vi "Transcriptor LabVIEW to C code Engine 2.vi"(7 "vi path":path, 8 "Error In":errorcluster, 11 "Diagram in":refnum<vi>) -> (0 "Error Out":errorcluster, 1 "output cluster":T1, 2 "transcripted code":string, 3 "Diagram out":refnum<vi>)   [LabVIEW 2014]
uses:
  types/LabVIEW Universal Transcriptor Cluster.ctl
panel:
  out "FiringOrder":string[](array[string])
  # "0. create definitions (ClusterConstant)\n1. get all wires and create their declarations\n2. if wires are connected to control or constant assign value to them\n3. translate elements of diagram by firing order\n4. assign values to outputs"
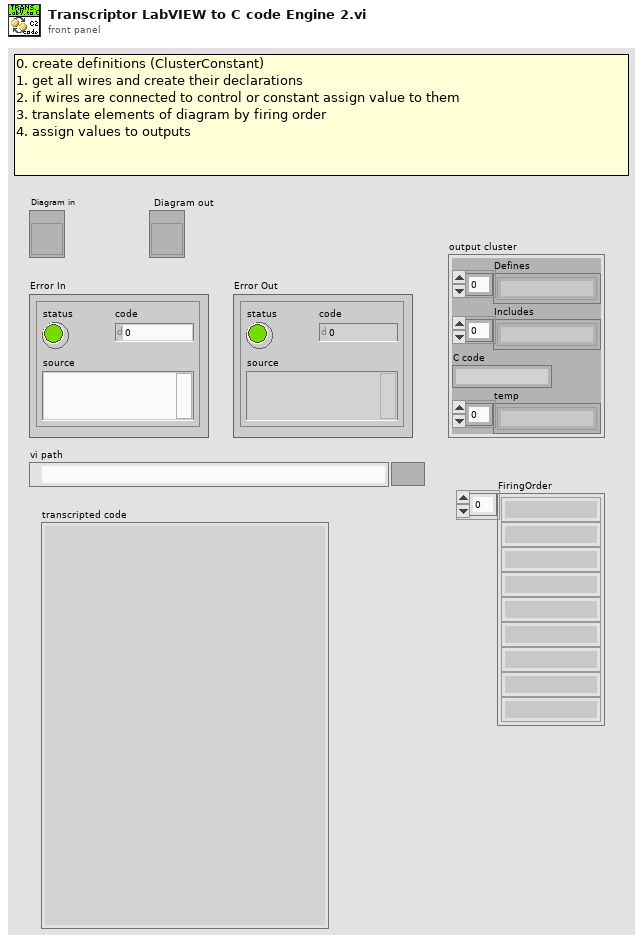
[diagram p1: front panel]
types:
  T1 = typedef "LabVIEW Universal Transcriptor Cluster.ctl" = cluster{"Defines":string[], "Includes":string[], "C code":string, "temp":string[]}
  T2 = cluster{"wire labels":string[], "wire terminals datatypes":string[][]}
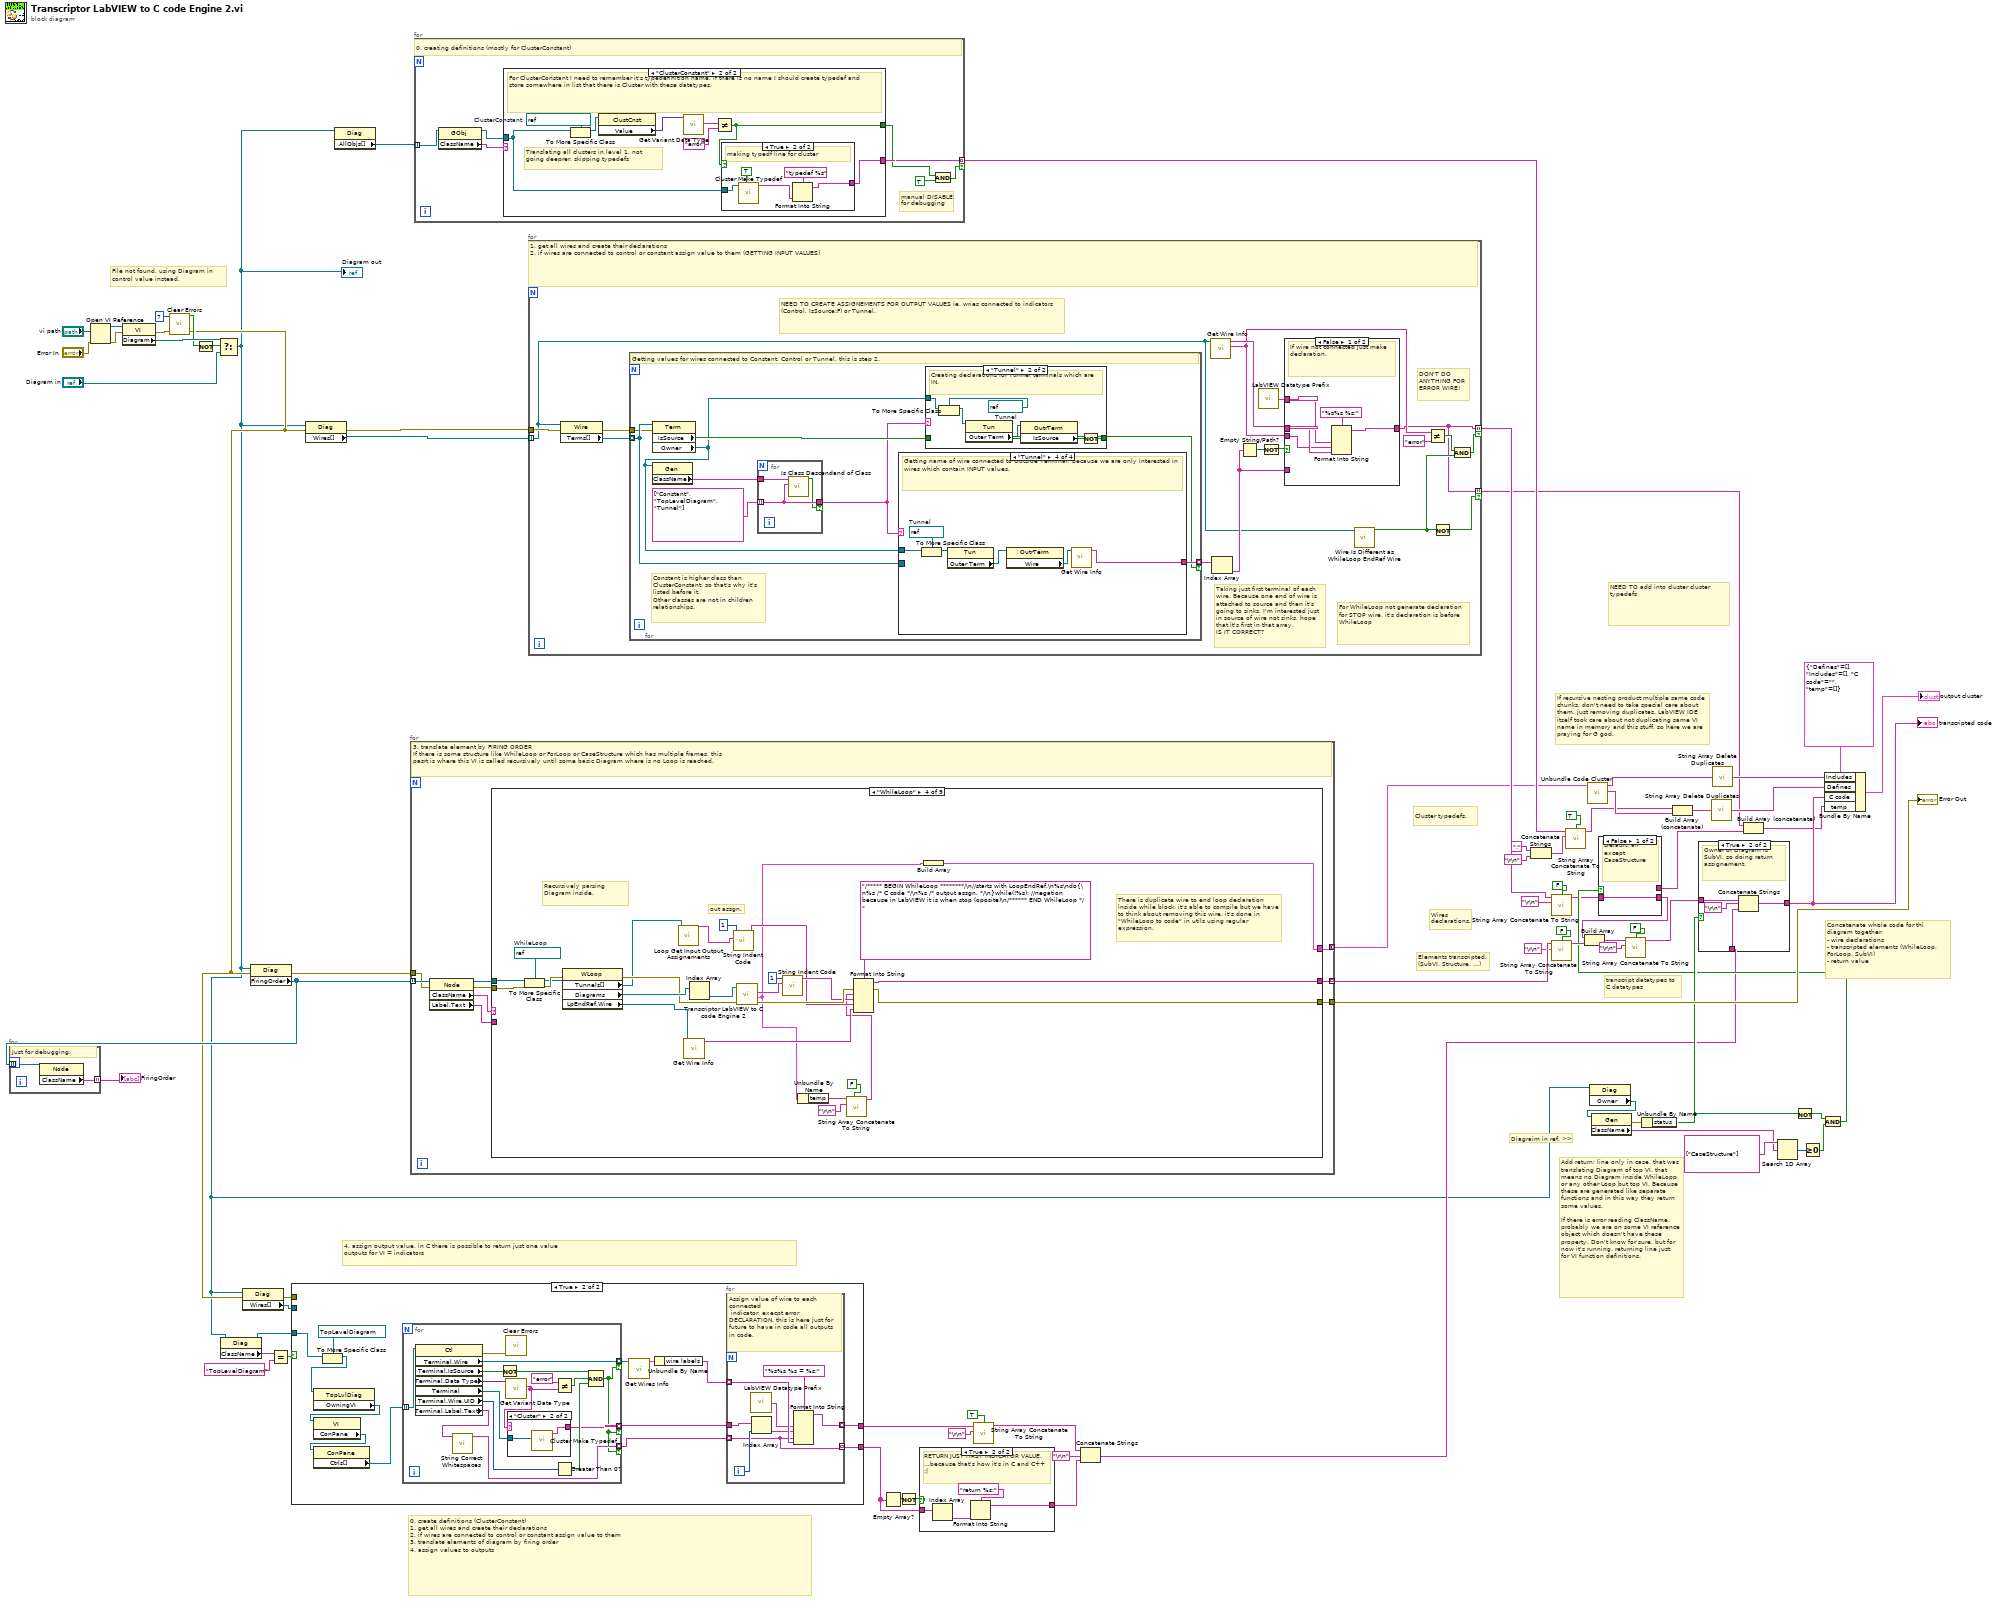
[diagram p0: block diagram]
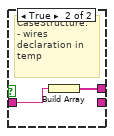
[diagram p7: hidden frame]
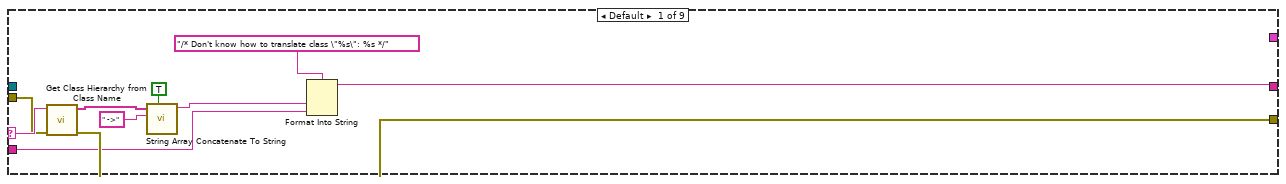
[diagram p9: hidden frame]
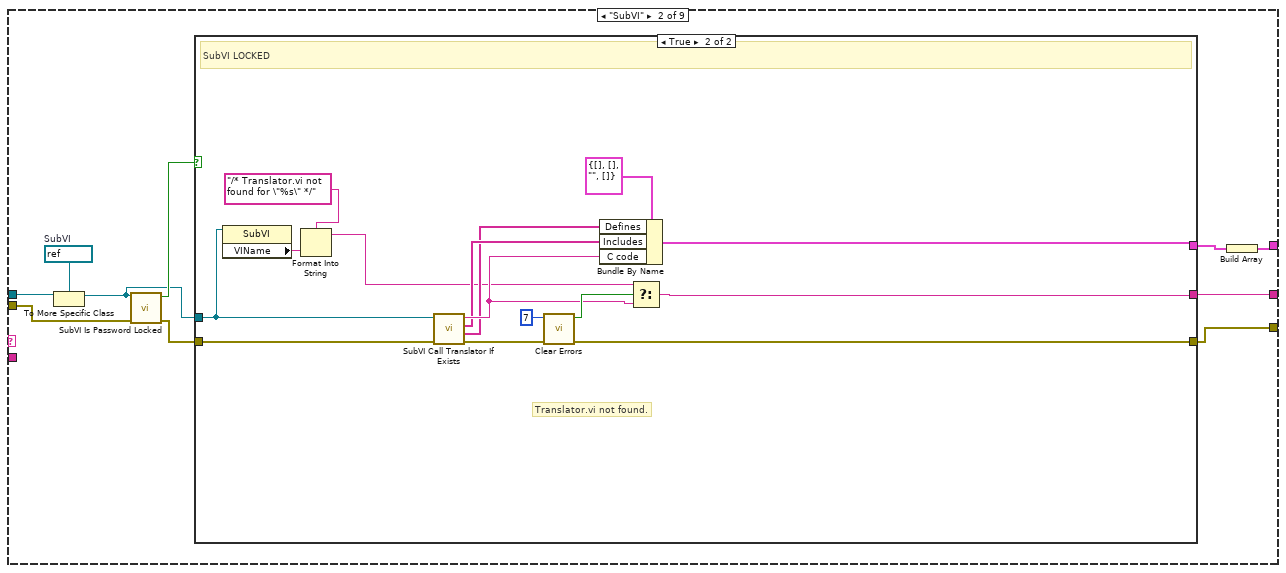
[diagram p10: hidden frame]
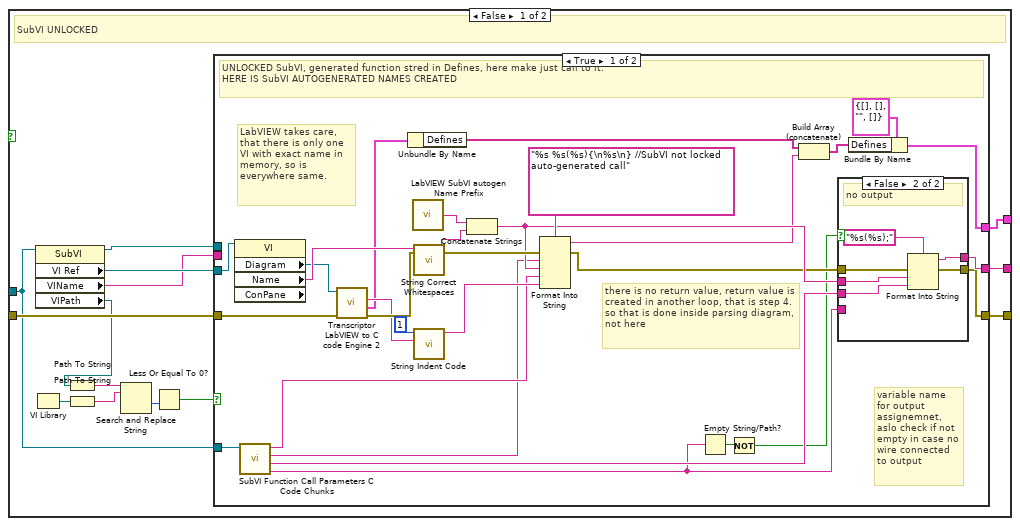
[diagram p11: hidden frame]
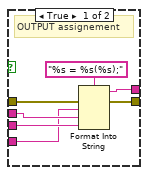
[diagram p12: hidden frame]
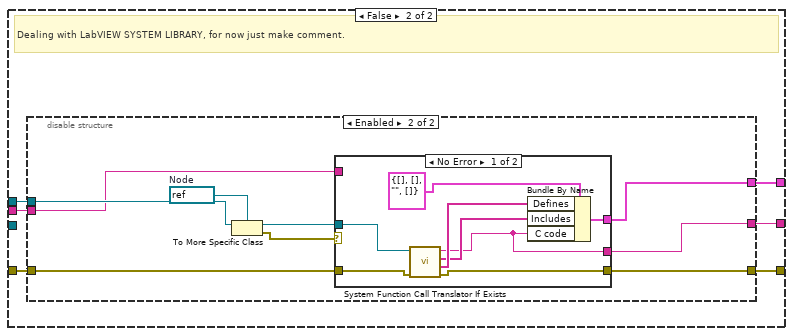
[diagram p13: hidden frame]
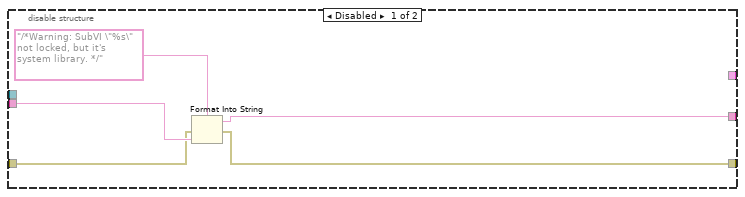
[diagram p14: hidden frame]
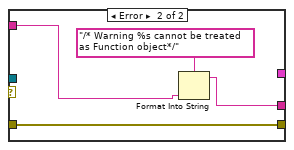
[diagram p15: hidden frame]
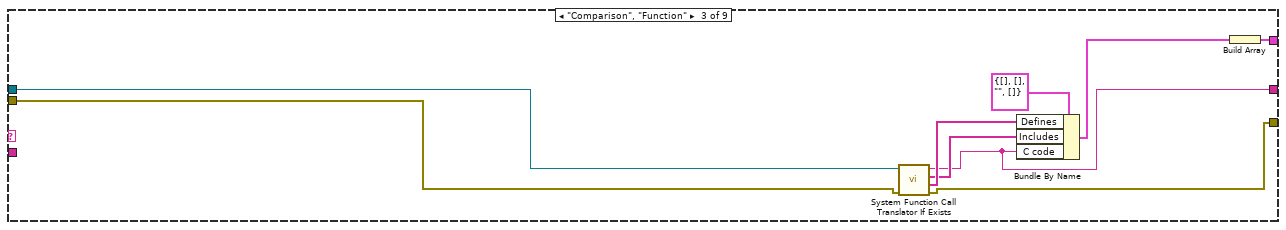
[diagram p16: hidden frame]
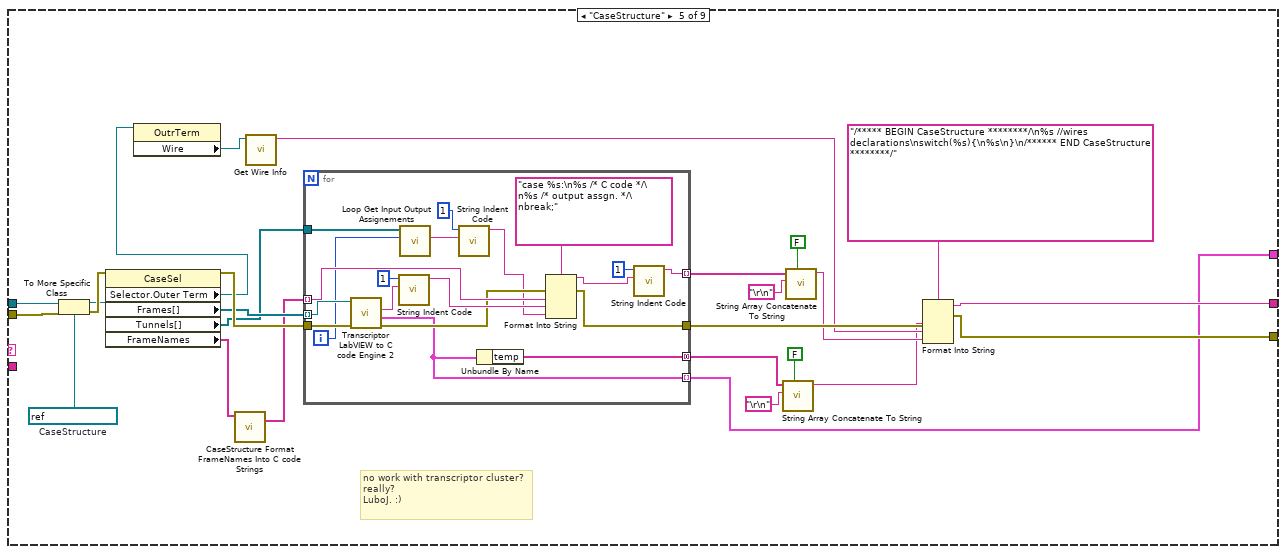
[diagram p17: hidden frame]
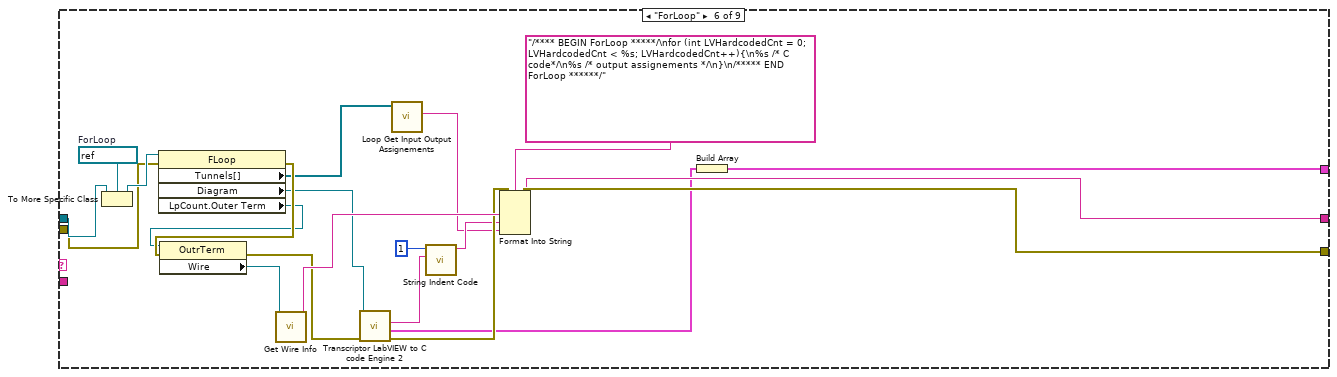
[diagram p18: hidden frame]
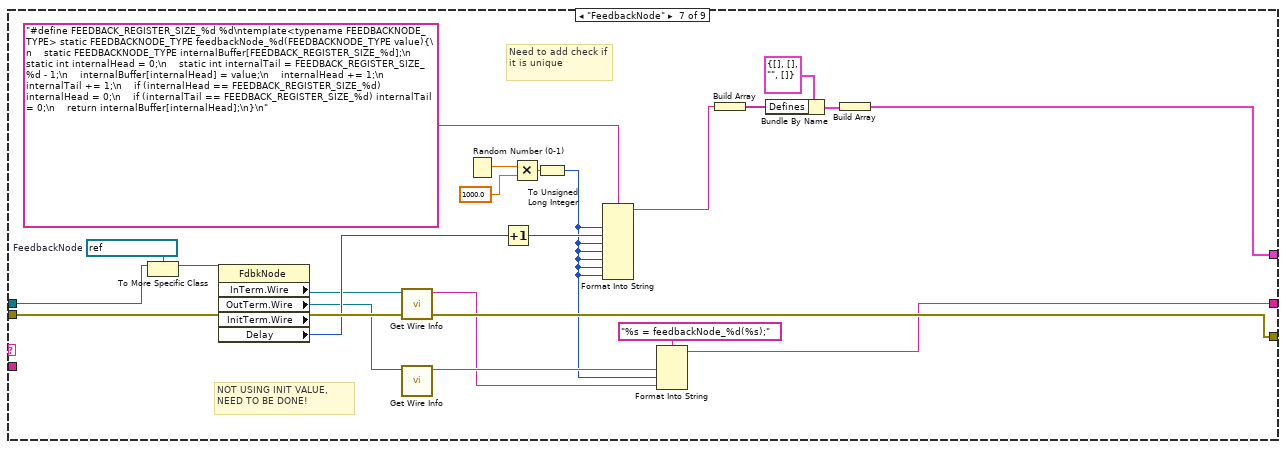
[diagram p19: hidden frame]
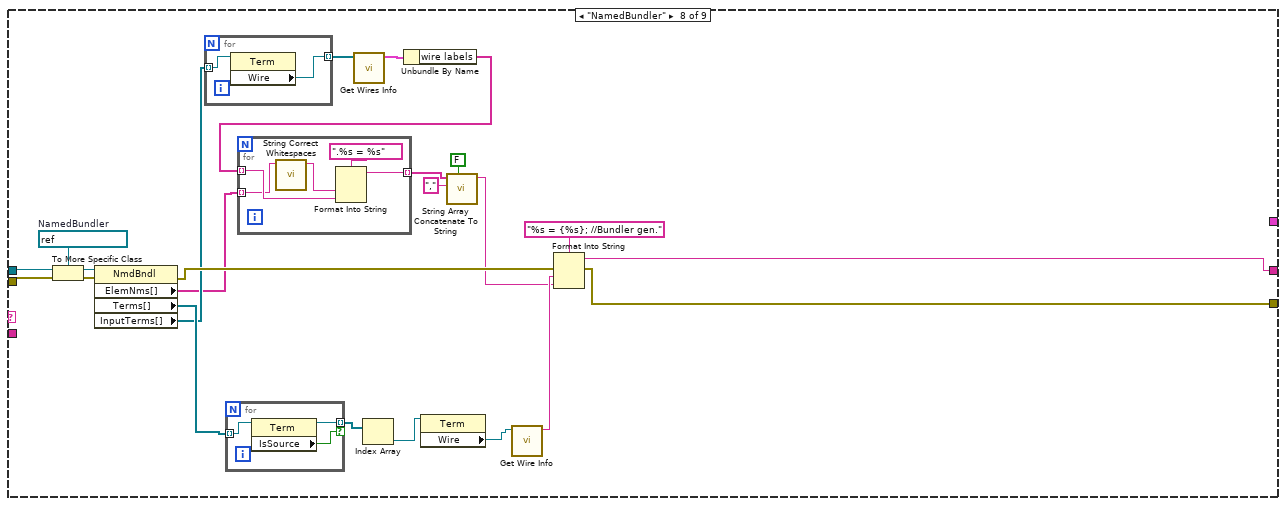
[diagram p20: hidden frame]
diagram:
  # "4. assign output value, in C there is possible to return just one value\noutputs for VI = indicators"
  # "Diagraim in ref. >>"
  # "Add return; line only in case, that was translating Diagram of top VI, that means no Diagram inside WhileLopp or any other Loop but top VI. Because these are generated like separate functions and in this way they return some values.\n\nIf there is error reading ClassName, probably we are on some VI reference object which doesn't have these property. Don't know for sure, but for now it's running, returning line just for VI function definitions."
  # "Concatenate whole code for thi diagram together:\n- wire declarations\n- transcripted elements (WhileLoop, ForLoop, SubVI)\n- return value"
  # "0. create definitions (ClusterConstant)\n1. get all wires and create their declarations\n2. if wires are connected to control or constant assign value to them\n3. translate elements of diagram by firing order\n4. assign values to outputs"
  # "If recursive nesting product multiple same code chunks, don't need to take special care about them, just removing duplicates, LabVIEW IDE itself took care about not duplicating same VI name in memory and this stuff, so here we are praying for G god."
  # "NEED TO add into cluster cluster typedefs"
  # "transcript datatypes to C datatypes"
  # "Elements transcripted.\n(SubVI, Structure, ...)"
  # "Wires declarations."
  # "Cluster typedefs."
  # "File not found, using Diagram in control value instead."
  n1 = Open VI Reference(vi path="vi path", error in (no error)="Error In") -> (vi reference=w20:refnum<vi>, error out=w74:errorcluster)  [unwired: 4 in]
  n2 = property class="VI"(reference=w20, error in=w74) -> (error out=w59:errorcluster, "Diagram"=w63:refnum<vi>)  [unwired: 1 out]
  n3 = call <vilib>:"Clear Errors.vi"("error in (no error)"=w59, "specific error code to clear (0: all)"=7) -> ("error out"=w42:errorcluster, "specific error cleared?"=w57:bool)  [unwired: 4 in]
  n4 = Not(x=w57) -> (.not. x?=w56:bool)
  n5 = Select(t=w63, s=w56, f="Diagram in") -> (s? t:f=w16:refnum<vi>)
  "Diagram out" <- w16
  n6 = property class="Diag"(reference=w16) -> (reference out=w15:refnum<vi>, "ClassName"=w18:string)  [unwired: 1 in, 1 out]
  n7 = property class="Diag"(reference=w16, error in=w42) -> (error out=w43:errorcluster, "Wires[]"=w44:refnum<vi>[])  [unwired: 1 out]
  n8 = property class="Diag"(reference=w16, error in=w42) -> (error out=w71:errorcluster, "FiringOrder"=w61:refnum<vi>[])  [unwired: 1 out]
  n9 = for {
    tunnel: w61 -> [w77] mode=indexing
    tunnel: [w76] -> w60 mode=indexing
    # "Just for debugging."
    n10 = property class="Node"(reference=w77) -> ("ClassName"=w76:string)  [unwired: 1 in, 2 out]
  }
  "FiringOrder" <- w60
  n11 = Equal?(x=w18, y="TopLevelDiagram" ("Parent ClassName")) -> (x = y?=w17:bool)
  n12 = case shown="True" w17 {
    tunnel: w44 -> [_ _]
    tunnel: w43 -> [_ _]
    tunnel: [_ w90] -> w39
    tunnel: [_ w89] -> w23
    tunnel: w15 -> [_ w87]
    frame False {
    }
    frame True {
      n13 = To More Specific Class(target class=refnum<vi> refnum, reference=w87) -> (specific class reference=w86:refnum<vi>)  [unwired: 1 in, 1 out]
      n14 = property class="TopLvlDiag"(reference=w86) -> ("OwningVI"=w85:refnum<vi>)  [unwired: 1 in, 2 out]
      n15 = property class="VI"(reference=w85) -> ("ConPane"=w84:refnum<vi>)  [unwired: 1 in, 2 out]
      n16 = property class="ConPane"(reference=w84) -> ("Ctrls[]"=w83:refnum<vi>[])  [unwired: 1 in, 2 out]
      n17 = for {
        tunnel: w83 -> [w106] mode=indexing
        tunnel: [w93] -> w82 mode=indexing if=w91
        tunnel: [w95] -> w81 mode=indexing if=w91
        tunnel: [w92] -> w80 mode=indexing if=w91
        n18 = property class="Ctl"(reference=w106) -> (error out=w105:errorcluster, "Terminal.Wire"=w92:refnum<vi>, "Terminal.IsSource"=w104:bool, "Terminal.Data Type"=w103:variant, "Terminal"=w100:refnum<vi>, "Terminal.Wire.UID"=w99:i32, "Terminal.Label.Text"=w94:string)  [unwired: 1 in, 1 out]
        n19 = call "String Correct Whitespaces.vi"("String in"=w94) -> ("String out"=w93:string)  [unwired: 10 in]
        n20 = Not(x=w104) -> (.not. x?=w98:bool)
        n21 = call <vilib>:"Clear Errors.vi"("error in (no error)"=w105) -> ()  [unwired: 5 in, 2 out]
        n22 = call "Get Variant Data Type.vi"("Variant in"=w103) -> ("first data type"=w101:string)  [unwired: 9 in, 1 out]
        n23 = case shown="\"Cluster\"" w101 {
          selector: w101 -> [w107 _]
          tunnel: [w107 w109] -> w95
          tunnel: w100 -> [_ w108]
          frame Default {
          }
          frame "Cluster" {
            n24 = call "Cluster Make Typedef.vi"("Terminal in"=w108) -> ("String"=w109:string)  [unwired: 10 in]
          }
        }
        n25 = Not Equal?(x="error", y=w101) -> (x != y?=w97:bool)
        n26 = Greater Than 0?(x=w99) -> (x > 0?=w96:bool)
        n27 = Compound Arithmetic op=AND(w98, w97, w96) -> (w91:bool)
      }
      n28 = call "Get Wires Info.vi"("connected\nwires refs."=w80) -> ("output cluster 2"=w79:T2)  [unwired: 10 in]
      n29 = Unbundle By Name(w79) -> ("wire labels"=w78:string[])
      n30 = for {
        tunnel: w82 -> [w110] mode=indexing
        tunnel: w78 -> [w115] mode=indexing
        tunnel: [w116] -> w90 mode=indexing
        tunnel: w81 -> [w113]
        tunnel: [w110] -> w89 mode=indexing
        i -> [w114]
        # "Assign value of wire to each connected\n indicator, execpt error\nDECLARATION, this is here just for future to have in code all outputs in code."
        n31 = call "LabVIEW Datatype Prefix.vi"() -> ("datatype prefix"=w111:string)
        n32 = Index Array(array=w113, index=w114) -> (element=w112:string)
        n33 = Format Into String(format string="%s%s %s = %s;", w111, w112, w110, w115) -> (resulting string=w116:string)  [unwired: 2 in, 1 out]
      }
    }
  }
  n34 = property class="Diag"(reference=w16, error in=w42) -> (error out=w72:errorcluster, "Wires[]"=w73:refnum<vi>[])  [unwired: 1 out]
  n35 = property class="Diag"(reference=w16) -> ("AllObjs[]"=w11:refnum<vi>[])  [unwired: 1 in, 2 out]
  n36 = for {
    tunnel: w61 -> [w126] mode=indexing
    tunnel: w71 -> [w124]
    tunnel: [w122] -> w70 mode=indexing
    tunnel: [w120] -> w32
    tunnel: [w119] -> w33 mode=concatenating
    # "3. translate element by FIRING ORDER\nIf there is some structure like WhileLoop or ForLoop or CaseStructure which has multiple frames, this\npasrt is where this VI is called recursively until some basic Diagram where is no Loop is reached."
    n37 = property class="Node"(reference=w126, error in=w124) -> (reference out=w123:refnum<vi>, error out=w121:errorcluster, "ClassName"=w125:string, "Label.Text"=w118:string)
    n38 = case shown="\"WhileLoop\"" w125 {
      selector: w125 -> [w134 _ _ _ _ _ _ _ _]
      tunnel: w123 -> [_ w146 w256 w284 w292 w350 w371 w395 w425]
      tunnel: [w135 w142 w253 w276 w305 w340 w359 w382 w406] -> w122
      tunnel: w121 -> [w129 w141 w257 w280 w308 w347 w372 w394 w424]
      tunnel: [w128 w139 w250 w274 w303 w341 w372 w380 w418] -> w120
      tunnel: [_ w137 w252 w263 w285 w330 w366 _ _] -> w119
      tunnel: w118 -> [w127 _ _ _ _ _ _ _ _]
      frame Default {
        n39 = call <vilib>:"Get Class Hierarchy from Class Name.vi"("error in (no error)"=w129, "Class Name"=w134) -> ("error out"=w128:errorcluster, "Class Hierarchy"=w132:string[])  [unwired: 8 in]
        n40 = call "String Array Concatenate To String.vi"("insert last delimiter?"=TRUE, "Delimiter char"=" ->", "Array String In"=w132) -> ("String"=w130:string)  [unwired: 8 in]
        n41 = Format Into String(format string="/* Don't know how to translate class \"%s\": %s */", w130, w127) -> (resulting string=w135:string)  [unwired: 2 in, 1 out]
      }
      frame "SubVI" {
        w145 = refnum<vi> refnum  # SubVI
        n42 = To More Specific Class(target class=w145, reference=w146) -> (specific class reference=w143:refnum<vi>)  [unwired: 1 in, 1 out]
        n43 = call "SubVI Is Password Locked.vi"("Error In"=w141, "SubVI ref"=w143) -> ("Error Out"=w140:errorcluster, "isPasswordLocked?"=w144:bool)  [unwired: 8 in]
        n44 = case shown="True" w144 {
          tunnel: w143 -> [w148 w239]
          tunnel: [w158 w245] -> w142
          tunnel: w140 -> [w160 w244]
          tunnel: [w157 w243] -> w139
          tunnel: [w149 w235] -> w138
          frame False {
            # "SubVI UNLOCKED"
            n45 = VI Library() -> (path=w154:path)
            n46 = property class="SubVI"(reference=w148) -> (reference out=w147:refnum<vi>, "VI Ref"=w159:refnum<vi>, "VIName"=w156:string, "VIPath"=w155:path)  [unwired: 1 in, 1 out]
            n47 = Path To String(path=w155) -> (string=w153:string)
            n48 = Path To String(path=w154) -> (string=w152:string)
            n49 = Search and Replace String(input string=w153, search string=w152) -> (number of replacements=w151:i32)  [unwired: 6 in, 3 out]
            n50 = Less Or Equal To 0?(x=w151) -> (x <= 0?=w150:bool)
            n51 = case shown="True" w150 {
              tunnel: w160 -> [w188 w205]
              tunnel: w159 -> [w172 _]
              tunnel: [w186 w207] -> w158
              tunnel: [w174 w204] -> w157
              tunnel: w156 -> [_ w206]
              tunnel: [w187 w202] -> w149
              tunnel: w148 -> [w170 _]
              tunnel: w147 -> [_ w203]
              frame True {
                # "variable name for output assignemnet, aslo check if not empty in case no wire connected to output"
                # "there is no return value, return value is created in another loop, that is step 4.\nso that is done inside parsing diagram, not here"
                # "LabVIEW takes care, that there is only one VI with exact name in memory, so is everywhere same."
                # "UNLOCKED SubVI, generated function stred in Defines, here make just call to it.\nHERE IS SubVI AUTOGENERATED NAMES CREATED"
                n52 = property class="VI" props=["Diagram", "Name", "ConPane"](reference=w172) -> ("Diagram"=w173:refnum<vi>, "Name"=w183:string)  [unwired: 1 in, 3 out]
                n53 = call "SubVI Function Call Parameters C Code Chunks.vi"("SubVI Refnum"=w170) -> ("SubVI output variable name"=w166:string, "SubVI func. params  declaration"=w168:string, "return datatype"=w164:string, "SubVI func. call params"=w169:string)  [unwired: 6 in, 1 out]
                n54 = call "Transcriptor LabVIEW to C code Engine 2.vi"("Error In"=w188, "Diagram in"=w173) -> ("Error Out"=w184:errorcluster, "output cluster"=w163:T1, "transcripted code"=w182:string)  [unwired: 6 in, 1 out]
                n55 = Unbundle By Name(w163) -> ("Defines"=w162:string[])
                n56 = call "LabVIEW SubVI autogen Name Prefix.vi"() -> ("datatype prefix"=w180:string)
                n57 = call "String Correct Whitespaces.vi"("String in"=w183) -> ("String out"=w179:string)  [unwired: 10 in]
                n58 = call "String Indent Code.vi"("complete code"=w182, "actual nested level"=1) -> ("indented code"=w171:string)  [unwired: 9 in]
                n59 = Concatenate Strings(w180, w179) -> (w178:string)
                n60 = Format Into String(format string="%s %s(%s){\n%s\n} //SubVI not locked auto-generated call", error in=w184, w164, w178, w169, w171) -> (resulting string=w176:string, error out=w175:errorcluster)  [unwired: 1 in]
                n61 = Empty String/Path?(string/path=w166) -> (empty?=w167:bool)
                n62 = Not(x=w167) -> (.not. x?=w165:bool)
                n63 = Build Array (concatenate)(w162, w176) -> (w177:string[])
                n64 = case shown="False" w165 {
                  tunnel: [w195 w201] -> w186
                  tunnel: w178 -> [w193 w199]
                  tunnel: w175 -> [w192 w198]
                  tunnel: [w191 w197] -> w174
                  tunnel: w168 -> [w190 w196]
                  tunnel: w166 -> [w189 _]
                  frame True {
                    # "OUTPUT assignement"
                    n65 = Format Into String(format string="%s = %s(%s);", error in=w192, w189, w193, w190) -> (resulting string=w195:string, error out=w191:errorcluster)  [unwired: 1 in]
                  }
                  frame False {
                    # "no output"
                    n66 = Format Into String(format string="%s(%s);", error in=w198, w199, w196) -> (resulting string=w201:string, error out=w197:errorcluster)  [unwired: 1 in]
                  }
                }
                n67 = Bundle By Name(cluster=T1 {"Defines"=[], "Includes"=[], "C code"="", "temp"=[]} ("input cluster"), "Defines"=w177) -> (w187:T1)
              }
              frame False {
                # "Dealing with LabVIEW SYSTEM LIBRARY, for now just make comment."
                n68 = disable-structure shown="Enabled" {
                  disable-tunnel: [w211 w216] -> w207
                  disable-tunnel: w206 -> [w210 w213]
                  disable-tunnel: w205 -> [w209 w215]
                  disable-tunnel: [w208 w221] -> w204
                  disable-tunnel: w203 -> [_ w220]
                  disable-tunnel: [_ w217] -> w202
                  frame Disabled {
                    n69 = Format Into String(format string="/*Warning: SubVI \"%s\" not locked, but it's system library. */", error in=w209, w210) -> (resulting string=w211:string, error out=w208:errorcluster)  [unwired: 1 in]
                  }
                  frame Enabled {
                    w219 = refnum<vi> refnum  # Node
                    n70 = To More Specific Class(target class=w219, reference=w220) -> (specific class reference=w218:refnum<vi>, error out=w214:errorcluster)  [unwired: 1 in]
                    n71 = case shown="No Error" w214 {
                      tunnel: [w229 w233] -> w221
                      tunnel: w218 -> [w228 _]
                      tunnel: [w225 _] -> w217
                      tunnel: [w224 w230] -> w216
                      tunnel: w215 -> [w223 w233]
                      tunnel: w213 -> [_ w231]
                      frame No Error {
                        n72 = call "System Function Call Translator If Exists.vi"("Error In"=w223, "Node Refnum"=w228) -> ("Error Out"=w229:errorcluster, "Defines"=w227:string[], "Includes"=w226:string[], "Replaced Code"=w224:string)  [unwired: 6 in]
                        n73 = Bundle By Name(cluster=T1 {"Defines"=[], "Includes"=[], "C code"="", "temp"=[]} ("input cluster"), "Defines"=w227, "Includes"=w226, "C code"=w224) -> (w225:T1)
                      }
                      frame Error {
                        n74 = Format Into String(format string="/* Warning %s cannot be treated as Function object*/" ("Replaced Code"), w231) -> (resulting string=w230:string)  [unwired: 2 in, 1 out]
                      }
                    }
                  }
                }
              }
            }
          }
          frame True {
            # "Translator.vi not found."
            # "SubVI LOCKED"
            n75 = property class="SubVI"(reference=w239) -> ("VIName"=w238:string)  [unwired: 1 in, 2 out]
            n76 = Format Into String(format string="/* Translator.vi not found for \"%s\" */" ("t"), w238) -> (resulting string=w236:string)  [unwired: 2 in, 1 out]
            n77 = call "SubVI Call Translator If Exists.vi"("Error In"=w244, "SubVI Refnum"=w239) -> ("Error Out"=w248:errorcluster, "Defines"=w240:string[], "Includes"=w241:string[], "Replaced Code"=w242:string)  [unwired: 6 in]
            n78 = call <vilib>:"Clear Errors.vi"("error in (no error)"=w248, "specific error code to clear (0: all)"=7) -> ("error out"=w243:errorcluster, "specific error cleared?"=w246:bool)  [unwired: 4 in]
            n79 = Bundle By Name(cluster=T1 {"Defines"=[], "Includes"=[], "C code"="", "temp"=[]} ("input cluster"), "Defines"=w240, "Includes"=w241, "C code"=w242) -> (w235:T1)
            n80 = Select(t=w236, s=w246, f=w242) -> (s? t:f=w245:string)
          }
        }
        n81 = Build Array(w138) -> (w137:T1[])
      }
      frame "Comparison", "Function" {
        n82 = call "System Function Call Translator If Exists.vi"("Error In"=w257, "Node Refnum"=w256) -> ("Error Out"=w250:errorcluster, "Defines"=w255:string[], "Includes"=w254:string[], "Replaced Code"=w253:string)  [unwired: 6 in]
        n83 = Bundle By Name(cluster=T1 {"Defines"=[], "Includes"=[], "C code"="", "temp"=[]} ("input cluster"), "Defines"=w255, "Includes"=w254, "C code"=w253) -> (w251:T1)
        n84 = Build Array(w251) -> (w252:T1[])
      }
      frame "WhileLoop" {
        w283 = refnum<vi> refnum  # WhileLoop
        # "out assgn."
        # "There is duplicate wire to end loop declaration inside while block, it's able to compile but we have to think about removing this wire, it's done in \"WhileLoop to code\" in utils using regular expression."
        # "Recursively parsing Diagram inside."
        n85 = To More Specific Class(target class=w283, reference=w284, error in=w280) -> (specific class reference=w273:refnum<vi>, error out=w282:errorcluster)
        n86 = property class="WLoop"(reference=w273, error in=w282) -> (error out=w279:errorcluster, "Tunnels[]"=w268:refnum<vi>[], "Diagrams"=w281:refnum<vi>[], "LpEndRef.Wire"=w272:refnum<vi>)  [unwired: 1 out]
        n87 = call "Loop Get Input Output Assignements.vi"("Loop Tunnels[]"=w268) -> ("Output assignements"=w265:string)  [unwired: 9 in, 1 out]
        n88 = call "Get Wire Info.vi"("Wire"=w272) -> ("wire label"=w267:string)  [unwired: 9 in, 1 out]
        n89 = Index Array(array=w281) -> (element=w278:refnum<vi>)  [unwired: 1 in]
        n90 = call "String Indent Code.vi"("complete code"=w265, "actual nested level"=1) -> ("indented code"=w264:string)  [unwired: 9 in]
        n91 = call "Transcriptor LabVIEW to C code Engine 2.vi"("Error In"=w279, "Diagram in"=w278) -> ("Error Out"=w275:errorcluster, "output cluster"=w262:T1, "transcripted code"=w271:string)  [unwired: 6 in, 1 out]
        n92 = call "String Indent Code.vi"("complete code"=w271, "actual nested level"=1) -> ("indented code"=w269:string)  [unwired: 9 in]
        n93 = Unbundle By Name(w262) -> ("temp"=w261:string[])
        n94 = call "String Array Concatenate To String.vi"("insert last delimiter?"=FALSE, "Delimiter char"="\r\n", "Array String In"=w261) -> ("String"=w258:string)  [unwired: 8 in]
        n95 = Format Into String(format string="/***** BEGIN WhileLoop ********/\n//starts with LoopEndRef.\n%s\ndo{\n%s /* C code */\n%s /* output assgn. */\n}while(!%s); //negation because in LabVIEW it is when stop (oposite)\n/****** END WhileLoop */", error in=w275, w258, w269, w264, w267) -> (resulting string=w276:string, error out=w274:errorcluster)  [unwired: 1 in]
        n96 = Build Array(w262) -> (w263:T1[])
      }
      frame "CaseStructure" {
        w310 = refnum<vi> refnum  # CaseStructure
        # "no work with transcriptor cluster? really?\nLuboJ. :)"
        n97 = To More Specific Class(target class=w310, reference=w292, error in=w308) -> (specific class reference=w302:refnum<vi>, error out=w309:errorcluster)
        n98 = property class="CaseSel"(reference=w302, error in=w309) -> (error out=w307:errorcluster, "Selector.Outer Term"=w300:refnum<vi>, "Frames[]"=w301:refnum<vi>[], "Tunnels[]"=w293:refnum<vi>[], "FrameNames"=w290:string[])  [unwired: 1 out]
        n99 = property class="OutrTerm"(reference=w300) -> ("Wire"=w299:refnum<vi>)  [unwired: 1 in, 2 out]
        n100 = call "CaseStructure Format FrameNames Into C code Strings.vi"("FrameNames in"=w290) -> ("c code cases names"=w291:string[])  [unwired: 10 in]
        n101 = call "Get Wire Info.vi"("Wire"=w299) -> ("wire label"=w298:string)  [unwired: 9 in, 1 out]
        n102 = for {
          tunnel: w307 -> [w329]
          tunnel: [w321] -> w304
          tunnel: w301 -> [w328] mode=indexing
          tunnel: w291 -> [w324] mode=indexing
          tunnel: [w319] -> w295 mode=indexing
          tunnel: w293 -> [w316]
          tunnel: [w312] -> w286 mode=concatenating
          tunnel: [w311] -> w285 mode=indexing
          i -> [w317]
          n103 = call "Transcriptor LabVIEW to C code Engine 2.vi"("Error In"=w329, "Diagram in"=w328) -> ("Error Out"=w322:errorcluster, "output cluster"=w311:T1, "transcripted code"=w326:string)  [unwired: 6 in, 1 out]
          n104 = call "String Indent Code.vi"("complete code"=w326, "actual nested level"=1) -> ("indented code"=w325:string)  [unwired: 9 in]
          n105 = call "Loop Get Input Output Assignements.vi"("Inside Terms[] offset"=w317, "Loop Tunnels[]"=w316) -> ("Output assignements"=w314:string)  [unwired: 8 in, 1 out]
          n106 = call "String Indent Code.vi"("complete code"=w314, "actual nested level"=1) -> ("indented code"=w313:string)  [unwired: 9 in]
          n107 = Unbundle By Name(w311) -> ("temp"=w312:string[])
          n108 = Format Into String(format string="case %s:\n%s /* C code */\n%s /* output assgn. */\nbreak;", error in=w322, w324, w325, w313) -> (resulting string=w318:string, error out=w321:errorcluster)  [unwired: 1 in]
          n109 = call "String Indent Code.vi"("complete code"=w318, "actual nested level"=1) -> ("indented code"=w319:string)  [unwired: 9 in]
        }
        n110 = call "String Array Concatenate To String.vi"("insert last delimiter?"=FALSE, "Delimiter char"="\r\n", "Array String In"=w286) -> ("String"=w287:string)  [unwired: 8 in]
        n111 = call "String Array Concatenate To String.vi"("insert last delimiter?"=FALSE, "Delimiter char"="\r\n", "Array String In"=w295) -> ("String"=w294:string)  [unwired: 8 in]
        n112 = Format Into String(format string="/***** BEGIN CaseStructure ********/\n%s //wires declarations\nswitch(%s){\n%s\n}\n/****** END CaseStructure ********/", error in=w304, w287, w298, w294) -> (resulting string=w305:string, error out=w303:errorcluster)  [unwired: 1 in]
      }
      frame "ForLoop" {
        w349 = refnum<vi> refnum  # ForLoop
        n113 = To More Specific Class(target class=w349, reference=w350) -> (specific class reference=w348:refnum<vi>)  [unwired: 1 in, 1 out]
        n114 = property class="FLoop"(reference=w348, error in=w347) -> (error out=w346:errorcluster, "Tunnels[]"=w333:refnum<vi>[], "Diagram"=w339:refnum<vi>, "LpCount.Outer Term"=w345:refnum<vi>)  [unwired: 1 out]
        n115 = property class="OutrTerm"(reference=w345, error in=w346) -> (error out=w338:errorcluster, "Wire"=w344:refnum<vi>)  [unwired: 1 out]
        n116 = call "Get Wire Info.vi"("Wire"=w344) -> ("wire label"=w342:string)  [unwired: 9 in, 1 out]
        n117 = call "Transcriptor LabVIEW to C code Engine 2.vi"("Error In"=w338, "Diagram in"=w339) -> ("Error Out"=w337:errorcluster, "output cluster"=w331:T1, "transcripted code"=w336:string)  [unwired: 6 in, 1 out]
        n118 = call "Loop Get Input Output Assignements.vi"("Loop Tunnels[]"=w333) -> ("Output assignements"=w332:string)  [unwired: 9 in, 1 out]
        n119 = call "String Indent Code.vi"("complete code"=w336, "actual nested level"=1) -> ("indented code"=w334:string)  [unwired: 9 in]
        n120 = Format Into String(format string="/**** BEGIN ForLoop *****/\nfor (int LVHardcodedCnt = 0;  LVHardcodedCnt < %s; LVHardcodedCnt++){\n%s /* C code*/\n%s /* output assignements */\n}\n/***** END ForLoop ******/", error in=w337, w342, w334, w332) -> (resulting string=w340:string, error out=w341:errorcluster)  [unwired: 1 in]
        n121 = Build Array(w331) -> (w330:T1[])
      }
      frame "FeedbackNode" {
        w369 = refnum<vi> refnum  # FeedbackNode
        # "Need to add check if it is unique"
        # "NOT USING INIT VALUE, NEED TO BE DONE!"
        n122 = To More Specific Class(target class=w369, reference=w371) -> (specific class reference=w370:refnum<vi>)  [unwired: 1 in, 1 out]
        n123 = property class="FdbkNode" props=["InTerm", "Wire", "OutTerm", "Wire", "InitTerm", "Wire", "Delay"](reference=w370) -> ("InTerm.Wire"=w363:refnum<vi>, "OutTerm.Wire"=w362:refnum<vi>, "Delay"=w368:i32)  [unwired: 1 in, 3 out]
        n124 = call "Get Wire Info.vi"("Wire"=w363) -> ("wire label"=w353:string)  [unwired: 9 in, 1 out]
        n125 = call "Get Wire Info.vi"("Wire"=w362) -> ("wire label"=w360:string)  [unwired: 9 in, 1 out]
        n126 = Random Number (0-1)() -> (number: 0 to 1=w357:dbl)
        n127 = Increment(x=w368) -> (x+1=w354:i32)
        n128 = Multiply(x=w357, y=1000.0) -> (x*y=w355:dbl)
        n129 = To Unsigned Long Integer(number=w355) -> (unsigned 32bit integer=w352:u32)
        n130 = Format Into String(format string="#define FEEDBACK_REGISTER_SIZE_%d %d\ntemplate<typename FEEDBACKNODE_TYPE> static FEEDBACKNODE_TYPE feedbackNode_%d(FEEDBACKNODE_TYPE value){\n    static FEEDBACKNODE_TYPE internalBuffer[FEEDBACK_REGISTER_SIZE_%d];\n    static int internalHead = 0;\n    static int internalTail = FEEDBACK_REGISTER_SIZE_%d - 1;\n    internalBuffer[internalHead] = value;\n    internalHead += 1;\n    internalTail += 1;\n    if (internalHead == FEEDBACK_REGISTER_SIZE_%d) internalHead = 0;\n    if (internalTail == FEEDBACK_REGISTER_SIZE_%d) internalTail = 0;\n    return internalBuffer[internalHead];\n}\n" ("Replaced Code"), w352, w354, w352, w352, w352, w352, w352) -> (resulting string=w364:string)  [unwired: 2 in, 1 out]
        n131 = Format Into String(format string="%s = feedbackNode_%d(%s);" ("Replaced Code"), w360, w352, w353) -> (resulting string=w359:string)  [unwired: 2 in, 1 out]
        n132 = Build Array(w364) -> (w365:string[])
        n133 = Bundle By Name(cluster=T1 {"Defines"=[], "Includes"=[], "C code"="", "temp"=[]} ("input cluster"), "Defines"=w365) -> (w367:T1)
        n134 = Build Array(w367) -> (w366:T1[])
      }
      frame "NamedBundler" {
        w392 = refnum<vi> refnum  # NamedBundler
        n135 = To More Specific Class(target class=w392, reference=w395, error in=w394) -> (specific class reference=w391:refnum<vi>, error out=w393:errorcluster)
        n136 = property class="NmdBndl"(reference=w391, error in=w393) -> (error out=w381:errorcluster, "ElemNms[]"=w377:string[], "Terms[]"=w387:refnum<vi>[], "InputTerms[]"=w379:refnum<vi>[])  [unwired: 1 out]
        n137 = for {
          tunnel: w379 -> [w402] mode=indexing
          tunnel: [w401] -> w378 mode=indexing
          n138 = property class="Term"(reference=w402) -> ("Wire"=w401:refnum<vi>)  [unwired: 1 in, 2 out]
        }
        n139 = for {
          tunnel: w387 -> [w405] mode=indexing
          tunnel: [w404] -> w386 mode=indexing if=w403
          n140 = property class="Term"(reference=w405) -> (reference out=w404:refnum<vi>, "IsSource"=w403:bool)  [unwired: 1 in, 1 out]
        }
        n141 = call "Get Wires Info.vi"("connected\nwires refs."=w378) -> ("output cluster 2"=w376:T2)  [unwired: 10 in]
        n142 = Index Array(array=w386) -> (element=w385:refnum<vi>)  [unwired: 1 in]
        n143 = Unbundle By Name(w376) -> ("wire labels"=w375:string[])
        n144 = for {
          tunnel: w377 -> [w397] mode=indexing
          tunnel: w375 -> [w399] mode=indexing
          tunnel: [w398] -> w374 mode=indexing
          n145 = call "String Correct Whitespaces.vi"("String in"=w397) -> ("String out"=w396:string)  [unwired: 10 in]
          n146 = Format Into String(format string=".%s = %s" ("Delimiter char"), w396, w399) -> (resulting string=w398:string)  [unwired: 2 in, 1 out]
        }
        n147 = property class="Term"(reference=w385) -> ("Wire"=w384:refnum<vi>)  [unwired: 1 in, 2 out]
        n148 = call "String Array Concatenate To String.vi"("insert last delimiter?"=FALSE, "Delimiter char"=",", "Array String In"=w374) -> ("String"=w373:string)  [unwired: 8 in]
        n149 = call "Get Wire Info.vi"("Wire"=w384) -> ("wire label"=w383:string)  [unwired: 9 in, 1 out]
        n150 = Format Into String(format string="%s = {%s}; //Bundler gen." ("Delimiter char"), error in=w381, w383, w373) -> (resulting string=w382:string, error out=w380:errorcluster)  [unwired: 1 in]
      }
      frame "NamedUnbundler" {
        w422 = refnum<vi> refnum  # NamedUnbundler
        # "Input structure name."
        n151 = To More Specific Class(target class=w422, reference=w425, error in=w424) -> (specific class reference=w421:refnum<vi>, error out=w423:errorcluster)
        n152 = property class="NmdUnbndl"(reference=w421, error in=w423) -> (error out=w419:errorcluster, "ElemNms[]"=w412:string[], "OutputTerms[]"=w414:refnum<vi>[], "Terms[]"=w417:refnum<vi>[])  [unwired: 1 out]
        n153 = for {
          tunnel: w417 -> [w438] mode=indexing
          tunnel: [w435] -> w416 mode=indexing if=w436
          n154 = property class="Term"(reference=w438) -> ("IsSource"=w437:bool, "Wire"=w435:refnum<vi>)  [unwired: 1 in, 2 out]
          n155 = Not(x=w437) -> (.not. x?=w436:bool)
        }
        n156 = for {
          tunnel: w414 -> [w434] mode=indexing
          tunnel: [w433] -> w413 mode=indexing
          n157 = property class="Term"(reference=w434) -> ("Wire"=w433:refnum<vi>)  [unwired: 1 in, 2 out]
        }
        n158 = call "Get Wires Info.vi"("connected\nwires refs."=w413) -> ("output cluster 2"=w411:T2)  [unwired: 10 in]
        n159 = Index Array(array=w416) -> (element=w415:refnum<vi>)  [unwired: 1 in]
        n160 = Unbundle By Name(w411) -> ("wire labels"=w410:string[])
        n161 = call "Get Wire Info.vi"("Wire"=w415) -> ("wire label"=w420:string)  [unwired: 9 in, 1 out]
        n162 = for {
          shift-right: [w429] -> w418
          shift-left: w419 -> [w430]
          tunnel: w420 -> [w428]
          tunnel: [w431] -> w409 mode=indexing
          tunnel: w412 -> [w427] mode=indexing
          tunnel: w410 -> [w426] mode=indexing
          n163 = Format Into String(format string="%s = %s.%s; //unbundle gen." ("Delimiter char"), error in=w430, w426, w428, w427) -> (resulting string=w431:string, error out=w429:errorcluster)  [unwired: 1 in]
        }
        n164 = call "String Array Concatenate To String.vi"("insert last delimiter?"=TRUE, "Delimiter char"="\r\n", "Array String In"=w409) -> ("String"=w406:string)  [unwired: 8 in]
      }
    }
  }
  "Error Out" <- w32
  n165 = for {
    tunnel: w11 -> [w445] mode=indexing
    tunnel: [w442] -> w49 mode=indexing if=w439
    # "manual DISABLE\nfor debugging"
    # "0. creating definitions (mostly for ClusterConstant)"
    n166 = property class="GObj"(reference=w445) -> (reference out=w443:refnum<vi>, "ClassName"=w444:string)  [unwired: 1 in, 1 out]
    n167 = case shown="\"ClusterConstant\"" w444 {
      tunnel: w443 -> [_ w447]
      tunnel: [_ w449] -> w442
      tunnel: [_ w448] -> w441
      frame Default {
        # "If wire is not wired to anything from what I have to read value, output is default Variant value (hope that is empty Variant), and there will be just wire declaration without assignement in generated code."
      }
      frame "ClusterConstant" {
        w450 = refnum<vi> refnum  # ClusterConstant
        # "Translating all clusters in level 1, not going deeprer, skipping typedefs"
        # "For ClusterConstant I need to remember it's typedefinition name, if there is no name I should create typedef and store somewhere in list that there is Cluster with these datatypes."
        n168 = To More Specific Class(target class=w450, reference=w447) -> (specific class reference=w446:refnum<vi>)  [unwired: 1 in, 1 out]
        n169 = property on="Property Node" class="ClustCnst"(reference=w446) -> ("Value"=w453:variant)  [unwired: 1 in, 2 out]
        n170 = call "Get Variant Data Type.vi"("Variant in"=w453) -> ("first data type"=w452:string)  [unwired: 9 in, 1 out]
        n171 = Not Equal?(x=w452, y="error") -> (x != y?=w448:bool)
        n172 = case shown="True" w448 {
          tunnel: w447 -> [_ w458]
          tunnel: [_ w455] -> w449
          frame False {
          }
          frame True {
            # "making typedf line for cluster"
            n173 = call "Cluster Make Typedef.vi"("skip first typedef?"=TRUE, "ClusterConstant refnum in"=w458) -> ("String"=w454:string)  [unwired: 9 in]
            n174 = Format Into String(format string="typedef %s", w454) -> (resulting string=w455:string)  [unwired: 2 in, 1 out]
          }
        }
      }
    }
    n175 = And(x=w441, y=TRUE) -> (x .and. y?=w439:bool)
  }
  n176 = for {
    tunnel: w73 -> [w462] mode=indexing
    tunnel: [w460] -> w65 mode=indexing if=w463
    tunnel: w72 -> [w468]
    tunnel: [w460] -> w1 mode=indexing if=w459
    # "For WhileLoop not generate declaration for STOP wire, it's declaration is before WhileLoop"
    # "Taking just first terminal of each wire. Because one end of wire is attached to source and then it's going to sinks, I'm interested just in source of wire not sinks, hope that it's first in that array.\nIS IT CORRECT?"
    # "NEED TO CREATE ASSIGNEMENTS FOR OUTPUT VALUES ie. wries connected to indicators (Control, IsSource:F) or Tunnel."
    # "DON'T DO ANYTHING FOR ERROR WIRE!"
    # "1. get all wires and create their declarations\n2. if wires are connected to control or constant assign value to them (GETTING INPUT VALUES)"
    n177 = property class="Wire"(reference=w462, error in=w468) -> (error out=w467:errorcluster, "Terms[]"=w475:refnum<vi>[])  [unwired: 1 out]
    n178 = for {
      tunnel: w475 -> [w494] mode=indexing
      tunnel: [w495] -> w474 mode=indexing if=w492
      tunnel: w467 -> [w493]
      # "Constant is higher class than ClusterConstant, so that's why it's listed before it.\nOther classes are not in children relationships."
      # "Getting values for wires connected to Constant, Control or Tunnel, this is step 2."
      n179 = property class="Term"(reference=w494, error in=w493) -> ("IsSource"=w491:bool, "Owner"=w490:refnum<vi>)  [unwired: 2 out]
      n180 = property class="Gen"(reference=w490) -> ("ClassName"=w488:string)  [unwired: 1 in, 2 out]
      n181 = for {
        tunnel: string[] ["Constant", "TopLevelDiagram", "Tunnel"] -> [w497] mode=indexing
        tunnel: w488 -> [w498]
        tunnel: [w497] -> w487 if=w496
        n182 = call "Is Class Descendand of Class.vi"("Parent ClassName"=w497, "ClassName"=w498) -> ("is Class descendant?"=w496:bool)  [unwired: 8 in, 1 out]
      }
      n183 = case shown="\"Tunnel\"" w487 {
        tunnel: w490 -> [_ _ w532 w537]
        tunnel: [_ w513 w529 w533] -> w495
        tunnel: w494 -> [_ w511 _ _]
        frame Default {
          # "If wire is not wired to anything from what I have to read value, output is default Variant value (hope that is empty Variant), and there will be just wire declaration without assignement in generated code."
        }
        frame "TopLevelDiagram" {
          w515 = refnum<vi> refnum  # ControlTerminal
          # "This is for wires connected to Control.\nNO indicator (it's just display value, not giving it to you)."
          n184 = To More Specific Class(target class=w515, reference=w511) -> (specific class reference=w514:refnum<vi>)  [unwired: 1 in, 1 out]
          n185 = property class="Term"(reference=w511) -> ("ClassName"=w510:string, "IsSource"=w506:bool)  [unwired: 1 in, 2 out]
          n186 = property class="CtrlTerm"(reference=w514) -> ("Control"=w509:refnum<vi>)  [unwired: 1 in, 2 out]
          n187 = Equal?(x="ControlTerminal", y=w510) -> (x = y?=w507:bool)
          n188 = And(x=w507, y=w506) -> (x .and. y?=w508:bool)
          n189 = case shown="True" w508 {
            tunnel: [_ w519] -> w513
            tunnel: w509 -> [_ w521]
            frame False {
              # "wire connected to indicator, do nothing"
            }
            frame True {
              # "wire connected to control, check if is on connector pane, if not use it's value"
              n190 = property class="Ctl"(reference=w521) -> ("Label.Text"=w520:string, "IsOnConPane"=w518:bool, "Value"=w517:variant, "Terminal"=w516:refnum<vi>)  [unwired: 1 in, 2 out]
              n191 = case shown="False" w518 {
                tunnel: w520 -> [_ w526]
                tunnel: [w523 w525] -> w519
                tunnel: w517 -> [w524 _]
                tunnel: w516 -> [w522 _]
                frame False {
                  # "This will not\nrun with\ncluster"
                  n192 = call "Get Variant Value.vi"("GObj Refnum"=w522, "Variant in"=w524) -> ("Variant value as string"=w523:string)  [unwired: 9 in]
                }
                frame True {
                  n193 = call "String Correct Whitespaces.vi"("String in"=w526) -> ("String out"=w525:string)  [unwired: 10 in]
                }
              }
            }
          }
        }
        frame "Constant" {
          w531 = refnum<vi> refnum  # Constant
          # "Add quotes for stirngs"
          # "Getting value of connected Constant. If it's String it's wrapped with quotes becuase whitespaces."
          n194 = To More Specific Class(target class=w531, reference=w532) -> (specific class reference=w530:refnum<vi>)  [unwired: 1 in, 1 out]
          n195 = property class="Const"(reference=w530) -> (reference out=w527:refnum<vi>, "Value"=w528:variant)  [unwired: 1 in, 1 out]
          n196 = call "Get Variant Value.vi"("GObj Refnum"=w527, "Variant in"=w528) -> ("Variant value as string"=w529:string)  [unwired: 9 in]
        }
        frame "Tunnel" {
          w538 = refnum<vi> refnum  # Tunnel
          # "Getting name of wire connected to Outside Terminal, because we are only interested in wires which contain INPUT values."
          n197 = To More Specific Class(target class=w538, reference=w537) -> (specific class reference=w536:refnum<vi>)  [unwired: 1 in, 1 out]
          n198 = property class="Tun"(reference=w536) -> ("Outer Term"=w535:refnum<vi>)  [unwired: 1 in, 2 out]
          n199 = property class="OutrTerm"(reference=w535) -> ("Wire"=w534:refnum<vi>)  [unwired: 1 in, 2 out]
          n200 = call "Get Wire Info.vi"("Wire"=w534) -> ("wire label"=w533:string)  [unwired: 9 in, 1 out]
        }
      }
      n201 = case shown="\"Tunnel\"" w487 {
        tunnel: [w499 w500] -> w492
        tunnel: w491 -> [w499 _]
        tunnel: w490 -> [_ w502]
        frame Default {
          # "For all others Terminal.Owner don't need to do anything else."
        }
        frame "Tunnel" {
          w504 = refnum<vi> refnum  # Tunnel
          # "Creating declarations for Tunnel terminals which are IN."
          n202 = To More Specific Class(target class=w504, reference=w502) -> (specific class reference=w505:refnum<vi>)  [unwired: 1 in, 1 out]
          n203 = property class="Tun"(reference=w505) -> ("Outer Term"=w503:refnum<vi>)  [unwired: 1 in, 2 out]
          n204 = property class="OutrTerm"(reference=w503) -> ("IsSource"=w501:bool)  [unwired: 1 in, 2 out]
          n205 = Not(x=w501) -> (.not. x?=w500:bool)
        }
      }
    }
    n206 = call "Get Wire Info.vi"("Wire"=w462) -> ("wire datatype"=w471:string, "wire label"=w472:string)  [unwired: 9 in]
    n207 = Index Array(array=w474) -> (element=w465:string)  [unwired: 1 in]
    n208 = Empty String/Path?(string/path=w465) -> (empty?=w473:bool)
    n209 = call "LabVIEW Datatype Prefix.vi"() -> ("datatype prefix"=w466:string)
    n210 = Not(x=w473) -> (.not. x?=w469:bool)
    n211 = case shown="False" w469 {
      tunnel: w472 -> [w478 w483]
      tunnel: w471 -> [w477 w482]
      tunnel: w465 -> [_ w485]
      tunnel: [w479 w484] -> w460
      tunnel: w466 -> [w476 w481]
      frame False {
        # "If wire not connected just make declaration."
        n212 = Format Into String(format string="%s%s %s;", w476, w477, w478) -> (resulting string=w479:string)  [unwired: 2 in, 1 out]
      }
      frame True {
        # "If wire connected to Constant or some value assign it."
        n213 = Format Into String(format string="%s%s %s = %s;", w481, w482, w483, w485) -> (resulting string=w484:string)  [unwired: 2 in, 1 out]
      }
    }
    n214 = call "Wire Is Different as WhileLoop EndRef Wire.vi"("Wire in"=w462) -> ("is different than WhileLoop endref?"=w461:bool)  [unwired: 10 in]
    n215 = Not Equal?(x=w471, y="error") -> (x != y?=w464:bool)
    n216 = Not(x=w461) -> (.not. x?=w459:bool)
    n217 = Compound Arithmetic op=AND(w464, w461) -> (w463:bool)
  }
  n218 = Empty Array?(array=w23) -> (empty?=w22:bool)
  n219 = Not(x=w22) -> (.not. x?=w21:bool)
  n220 = case shown="True" w21 {
    tunnel: [_ w540] -> w36
    tunnel: w23 -> [_ w539]
    frame False {
    }
    frame True {
      # "RETURN JUST FIRST INDICATOR VALUE.\n...because that's how it's in C and C++ :|"
      n221 = Index Array(array=w539) -> (element=w541:string)  [unwired: 1 in]
      n222 = Format Into String(format string="return %s;", w541) -> (resulting string=w540:string)  [unwired: 2 in, 1 out]
    }
  }
  n223 = call "String Array Concatenate To String.vi"("insert last delimiter?"=TRUE, "Delimiter char"="\r\n", "Array String In"=w39) -> ("String"=w37:string)  [unwired: 8 in]
  n224 = Concatenate Strings(w37, "\r\n", w36) -> (w24:string)
  n225 = Concatenate Strings(";" ("string"), "\r\n") -> (w12:string)
  n226 = call "String Array Concatenate To String.vi"("insert last delimiter?"=FALSE, "Delimiter char"="\r\n", "Array String In"=w65) -> ("String"=w26:string)  [unwired: 8 in]
  n227 = call "String Array Concatenate To String.vi"("insert last delimiter?"=FALSE, "Delimiter char"="\r\n", "Array String In"=w70) -> ("String"=w64:string)  [unwired: 8 in]
  n228 = call "String Array Concatenate To String.vi"("insert last delimiter?"=TRUE, "Delimiter char"=w12, "Array String In"=w49) -> ("String"=w6:string)  [unwired: 8 in]
  n229 = call "Unbundle Code Cluster.vi"("code chunks cluster"=w33) -> ("Defines"=w45:string[], "Includes"=w5:string[])  [unwired: 8 in, 1 out]
  n230 = property class="Diag"(reference=w16) -> ("Owner"=w31:refnum<vi>)  [unwired: 1 in, 2 out]
  n231 = property class="Gen"(reference=w31) -> (error out=w30:errorcluster, "ClassName"=w9:string)  [unwired: 1 in, 1 out]
  n232 = Unbundle By Name(w30) -> ("status"=w29:bool)
  n233 = Build Array (concatenate)(w6, w45) -> (w46:string[])
  n234 = call "String Array Delete Duplicates.vi"("Array"=w46) -> ("Output array"=w47:string[])
  n235 = call "String Array Delete Duplicates.vi"("Array"=w5) -> ("Output array"=w48:string[])
  n236 = Search 1D Array(1D array=string[] ["CaseStructure"], element=w9) -> (index of element=w8:i32)  [unwired: 1 in]
  n237 = Not(x=w29) -> (.not. x?=w28:bool)
  n238 = Greater Or Equal To 0?(x=w8) -> (x >= 0?=w7:bool)
  n239 = And(x=w28, y=w7) -> (x .and. y?=w27:bool)
  n240 = case shown="False" w27 {
    tunnel: w26 -> [w543 w545]
    tunnel: [w543 _] -> w25
    tunnel: [_ w544] -> w3
    frame False {
      # "Default, all except CaseStructure"
    }
    frame True {
      # "CaseStructure:\n- wires declaration in temp"
      n241 = Build Array(w545) -> (w544:string[])
    }
  }
  n242 = Build Array(w25, w64) -> (w54:string[])
  n243 = call "String Array Concatenate To String.vi"("insert last delimiter?"=FALSE, "Delimiter char"="\r\n", "Array String In"=w54) -> ("String"=w35:string)  [unwired: 8 in]
  n244 = case shown="True" w29 {
    tunnel: w35 -> [w546 w550]
    tunnel: [w546 w549] -> w34
    tunnel: w24 -> [_ w548]
    frame False {
      # "Owner of Diagram is Loop or something else, don't do retur ...; assignement."
    }
    frame True {
      # "Owner of Diagram is SubVI, so doing return assignement."
      n245 = Concatenate Strings(w550, "\r\n", w548) -> (w549:string)
    }
  }
  "transcripted code" <- w34
  n246 = Build Array (concatenate)(w1, w3) -> (w2:string[])
  n247 = Bundle By Name(cluster=T1 {"Defines"=[], "Includes"=[], "C code"="", "temp"=[]} ("input cluster"), "Includes"=w48, "Defines"=w47, "C code"=w34, "temp"=w2) -> (→"output cluster":T1)
